vi "Add Resource.vi"(7 "TagPrefix":string, 8 "error in (no error)":errorcluster, 9 "ItemText":string, 10 "ItemName":string, 11 "GObject in":refnum<class "GObject.lvclass">) -> (0 "error out":errorcluster, 3 "GObject out":refnum<class "GObject.lvclass">)   [LabVIEW 2013, in "SET Project Data.lvlib" / "GObject.lvclass"]
uses:
  GObject.lvclass
  GObject.lvclass/GObject.ctl
  Resource Data Class/Resource Data.lvclass
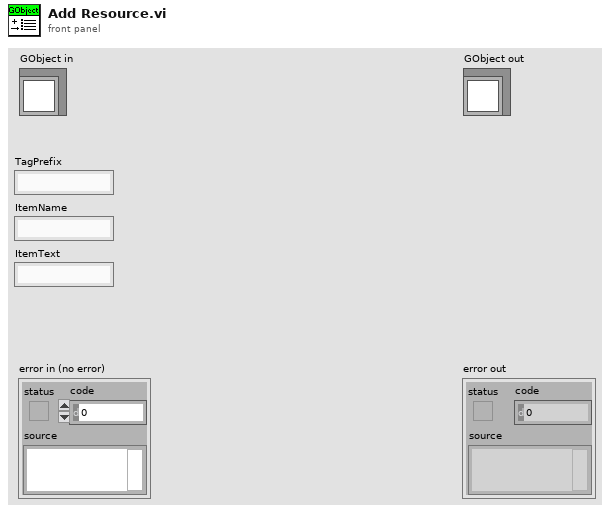
[diagram p1: front panel]
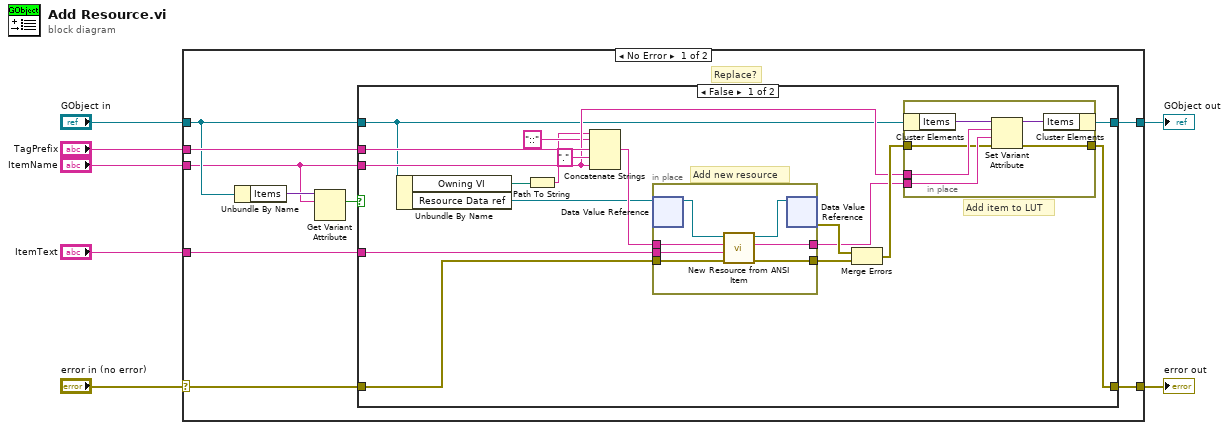
[diagram p0: block diagram]
diagram:
  n1 = case shown="No Error" "error in (no error)" {
    selector: "error in (no error)" -> [w15 w50]
    tunnel: [w14 w50] -> w6
    tunnel: [w13 w49] -> w4
    tunnel: "GObject in" -> [w11 w49]
    tunnel: "TagPrefix" -> [w16 _]
    tunnel: "ItemName" -> [w9 _]
    tunnel: "ItemText" -> [w12 _]
    frame No Error {
      # "Replace?"
      n2 = Unbundle By Name(w11) -> ("Items"=w10:variant)
      n3 = Get Variant Attribute(Variant=w10, name=w9) -> (found=w8:bool)  [unwired: 2 in, 3 out]
      n4 = case shown="False" w8 {
        tunnel: w16 -> [w31 _]
        tunnel: w15 -> [w30 w47]
        tunnel: [w20 w47] -> w14
        tunnel: [w24 w48] -> w13
        tunnel: w12 -> [w29 _]
        tunnel: w11 -> [w21 w48]
        tunnel: w9 -> [w23 _]
        frame False {
          # "Add item to LUT"
          # "Add new resource"
          n5 = Unbundle By Name(w21) -> ("Owning VI"=w19:path, "Resource Data ref"=w28:refnum<data-value>)
          n6 = Path To String(path=w19) -> (string=w17:string)
          n7 = Concatenate Strings(w17, "::" ("string"), w31, "." ("string"), w23) -> (w32:string)
          n8 = in-place {
            in-place-border: [w46] -> w22
            in-place-border: [w45] -> w27
            in-place-border: w32 -> [w44]
            in-place-border: w30 -> [w43]
            in-place-border: w29 -> [w42]
            n9 = in-place-dvr #1(w28) -> (w41:refnum<class "Resource Data.lvclass">)  [unwired: 1 out]
            n10 = call "New Resource from ANSI Item.vi"("error in (no error)"=w43, "Default String (ANSI)"=w42, "Tag (ANSI)"=w44, "LangFile in"=w41) -> ("error out"=w45:errorcluster, "RID"=w46:string, "LangFile out"=w40:refnum<class "Resource Data.lvclass">)  [unwired: 5 in]
            n11 = in-place-dvr #1(w40) -> (w26:errorcluster)  [unwired: 1 out]
          }
          n12 = Merge Errors(w26, w27) -> (w25:errorcluster)
          n13 = in-place {
            in-place-border: w23 -> [w39]
            in-place-border: w22 -> [w38]
            in-place-border: w25 -> [w35]
            in-place-border: [w34] -> w20
            n14 = in-place-cluster #2(w21) -> ("Items"=w37:variant)
            n15 = Set Variant Attribute(Variant=w37, name=w39, value=w38, error in=w35) -> (Variant out=w36:variant, error out=w34:errorcluster)  [unwired: 1 out]
            n16 = in-place-cluster #2("Items"=w36) -> (w24:refnum<class "GObject.lvclass">)
          }
        }
        frame True {
          # "#TODO - Handle item update case"
        }
      }
    }
    frame Error {
    }
  }
  "error out" <- w6
  "GObject out" <- w4
